vi "Init Screen.vi"(8 "error in":errorcluster) -> (0 "error out":errorcluster)   [LabVIEW 2020, in "Panther Dashboard.lvlib"]
uses:
  Panther Dashboard.lvlib
  Controls/Search.ctl
  Controls/Listbox.ctl
  Controls/Open Project.ctl
  Class/Project/Project.lvclass
panel:
  in  "Projects Opened":T1
  in  "Targets":T1
  out "Current Selection":string
  in  "Scan All":bool caption="Checkbox"
  in  "Include Dependencies":bool caption="Checkbox"
  in  "Scan Project":T2
  in  "Project history":T1
  in  "Open DQMH Project":T3
  # "Scanning a Project\n1. Select the Project and Target  where you want to work with Panther Dashboard\n2. Choose whether to scan the entire project or select specific modules to scan.\n3. Decide whether to include dependency modules in the scan.\n4. Click the Scan Project button."
  # "Working with previously Scanned Projects (Listed in Project History List):\n1. Double Click one of the Projects listed in the Project History\n\nWorking with previously Scanned Projects (not listed in the Project History)\n2. Click the Open DQMH Project and browse for your previously Scanned Project"
  # "1"
  # "1"
  # "1"
  # "2"
  # "4"
  # "2"
  # "3"
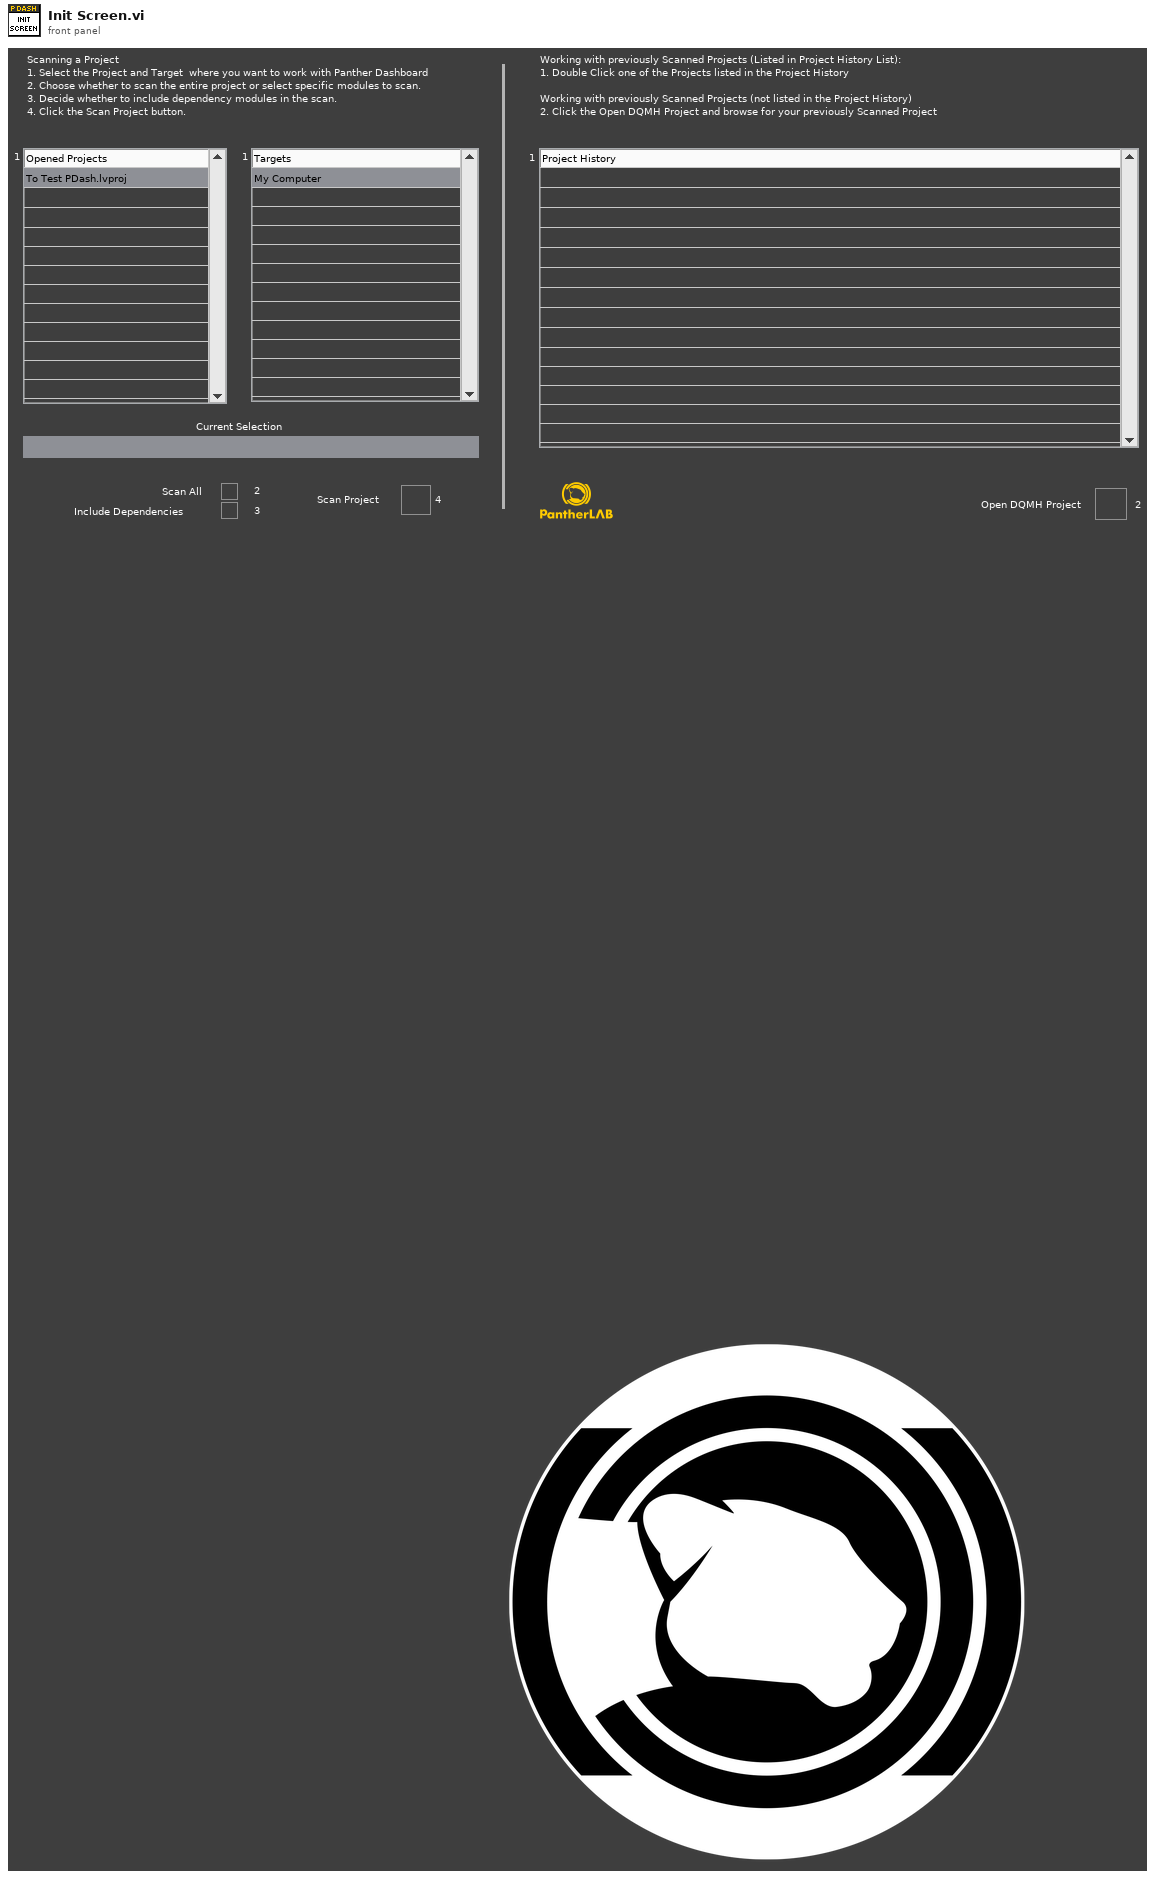
[diagram p1: front panel]
types:
  T1 = typedef "Listbox.ctl" = i32
  T2 = typedef "Search.ctl" = bool
  T3 = typedef "Open Project.ctl" = bool
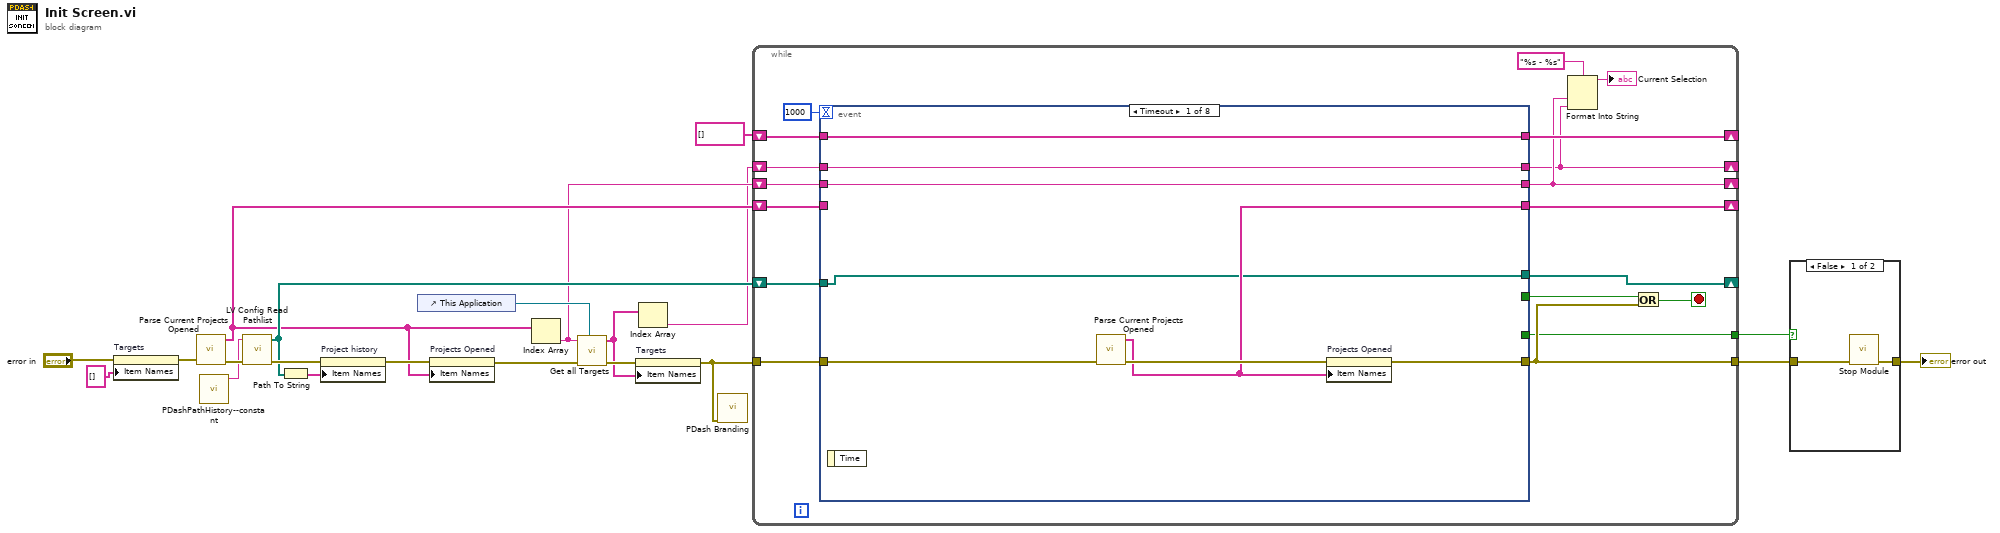
[diagram p0: block diagram]
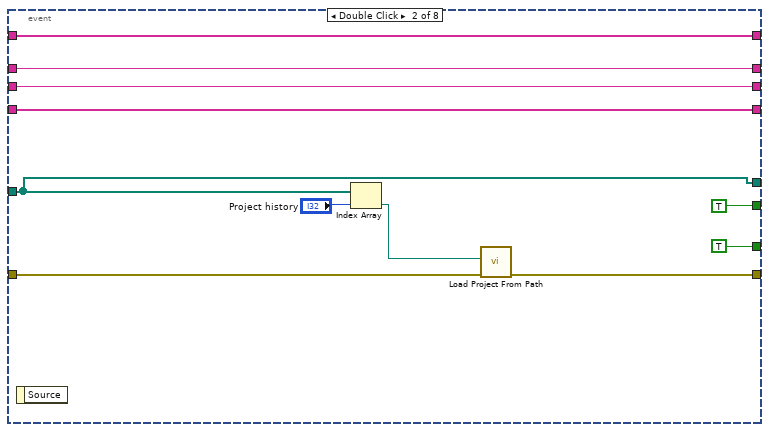
[diagram p2: hidden frame]
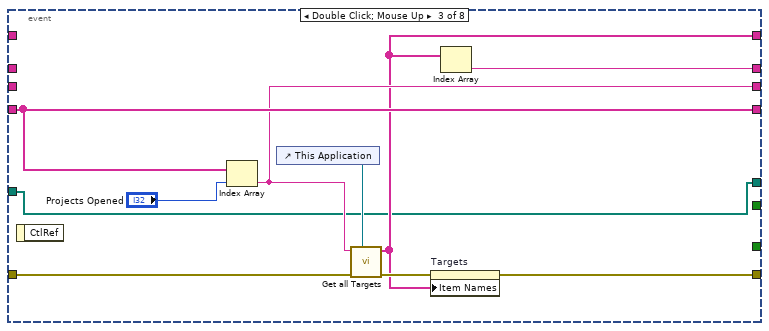
[diagram p3: hidden frame]
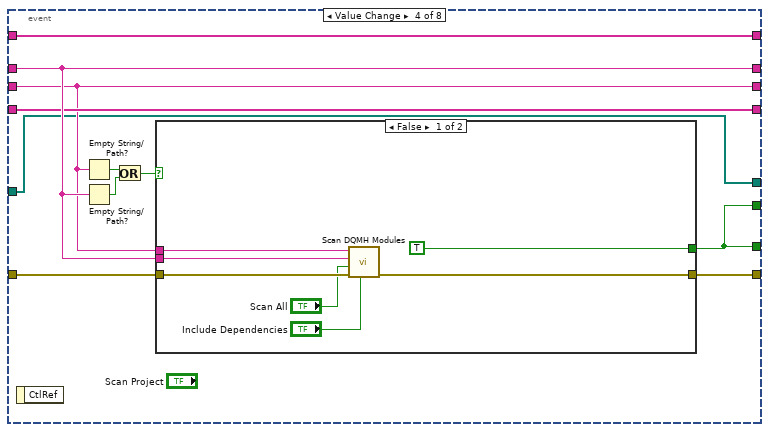
[diagram p4: hidden frame]
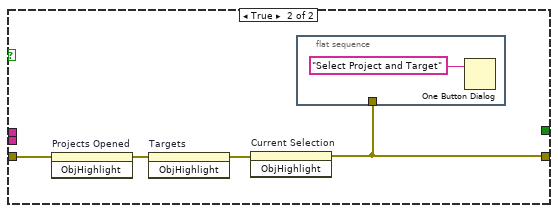
[diagram p5: hidden frame]
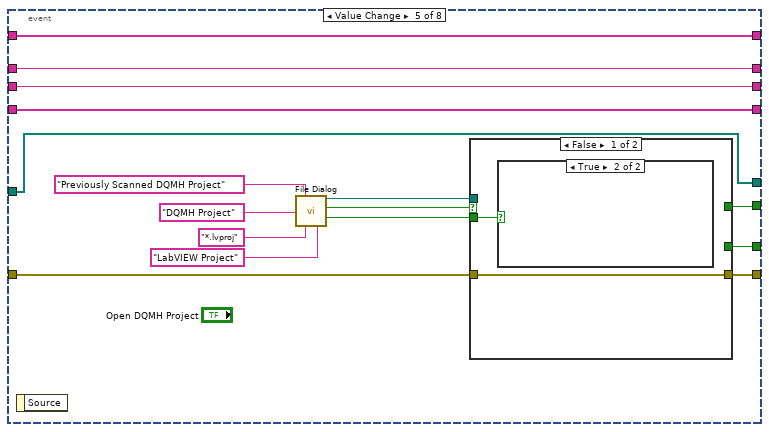
[diagram p6: hidden frame]
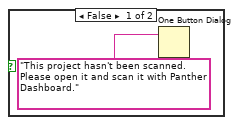
[diagram p7: hidden frame]
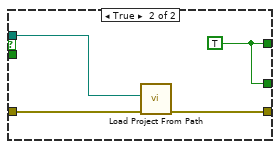
[diagram p8: hidden frame]
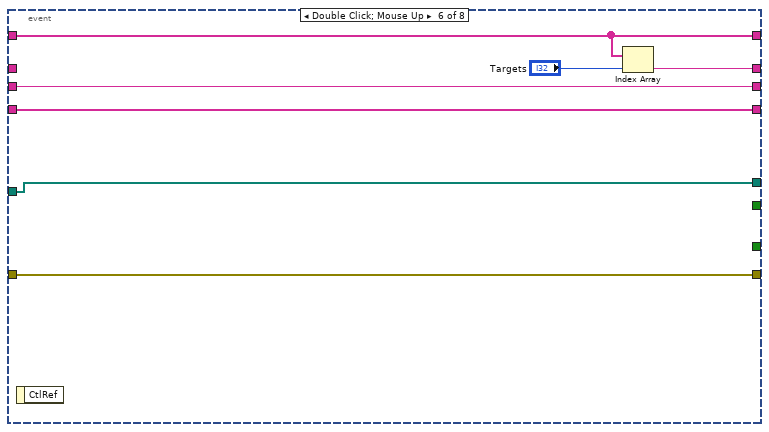
[diagram p9: hidden frame]
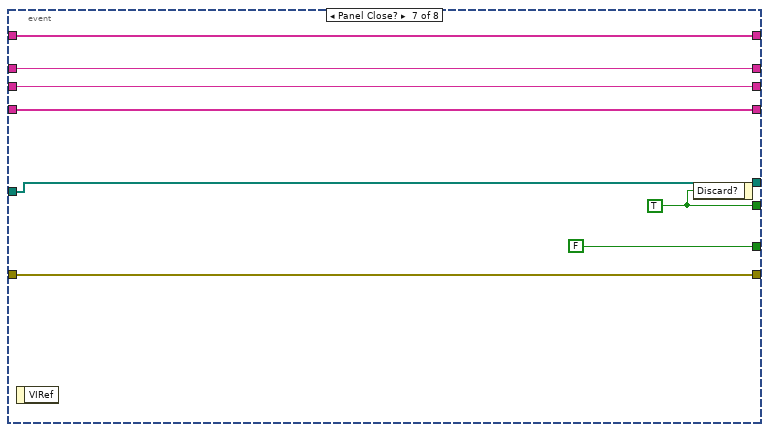
[diagram p10: hidden frame]
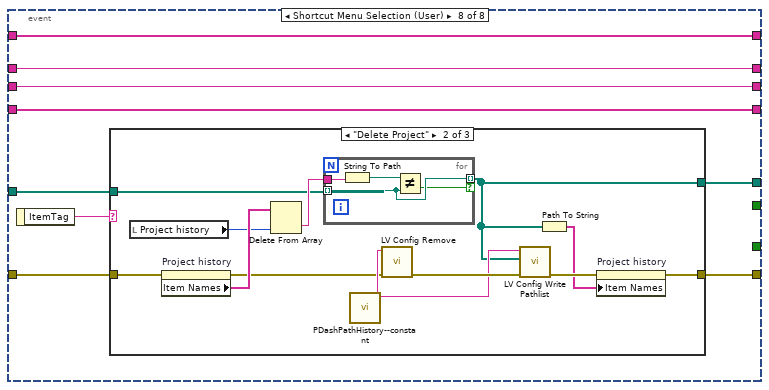
[diagram p11: hidden frame]
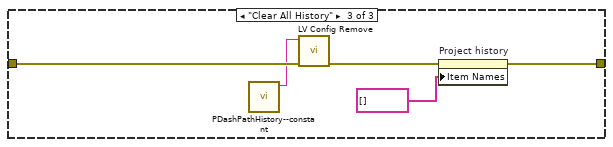
[diagram p13: hidden frame]
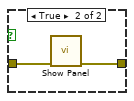
[diagram p14: hidden frame]
diagram:
  n1 = property on="Targets" class="LstBox (strict)"(error in="error in", "Item Names"=string[] []) -> (error out=w17:errorcluster)  [unwired: 1 in, 1 out]
  n2 = call "Parse Current Projects Opened.vi"("error in"=w17) -> ("error out"=w20:errorcluster, "Current Projects Opened"=w5:string[])  [unwired: 9 in]
  n3 = call "PDashPathHistory--constant.vi"() -> ("PDashPathHistory"=w12:string)  [unwired: 11 in]
  n4 = call <resource>:"LV Config Read Pathlist.vi"("error in"=w20, "key"=w12) -> ("error out"=w19:errorcluster, "value"=w11:path[])  [unwired: 3 in, 1 out]
  n5 = Path To String(path=w11) -> (string=w1:string[])
  n6 = property on="Project history" class="LstBox (strict)"(error in=w19, "Item Names"=w1) -> (error out=w18:errorcluster)  [unwired: 1 in, 1 out]
  n7 = control-ref of="This Application"() -> (w7:refnum<vi>)
  n8 = property on="Projects Opened" class="LstBox (strict)"(error in=w18, "Item Names"=w5) -> (error out=w14:errorcluster)  [unwired: 1 in, 1 out]
  n9 = Index Array(array=w5) -> (element=w4:string)  [unwired: 1 in]
  n10 = call "Get all Targets.vi"("App instance"=w7, "error in"=w14, "Project Selection"=w4) -> ("error out"=w15:errorcluster, "Targets"=w3:string[])  [unwired: 7 in]
  n11 = property on="Targets" class="LstBox (strict)"(error in=w15, "Item Names"=w3) -> (error out=w6:errorcluster)  [unwired: 1 in, 1 out]
  n12 = Index Array(array=w3) -> (element=w2:string)  [unwired: 1 in]
  n13 = call "PDash Branding.vi"("error in"=w6) -> ()  [unwired: 11 in]
  n14 = while {
    shift-right: [w34] -> _
    shift-left: string[] [] ("Targets") -> [w33]
    shift-right: [w25] -> _
    shift-left: w2 -> [w32]
    shift-right: [w26] -> _
    shift-left: w4 -> [w31]
    tunnel: [w28] -> w8
    shift-right: [w27] -> _
    shift-left: w5 -> [w35]
    tunnel: w6 -> [w39]
    tunnel: [w38] -> w21
    shift-right: [w23] -> _
    shift-left: w11 -> [w37]
    stop <- w29 stop-if-true
    n15 = event shown="[0] Timeout" {
      selector: _ -> [_ _ _ _ _ _ _ _]
      dyn-events: _ -> [_ _ _ _ _ _ _ _]
      timeout: 1000 -> [_ _ _ _ _ _ _ _]
      tunnel: w39 -> [w47 w58 w68 w79 w106 w121 w129 w138]
      tunnel: [w45 w57 w66 w78 w107 w121 w129 w137] -> w38
      tunnel: w37 -> [w40 w56 w59 w69 w92 w115 w122 w132]
      tunnel: [_ TRUE ("Discard?") _ w74 w101 _ w128 _] -> w36
      tunnel: w35 -> [_ w48 w65 w72 w102 w116 w123 w131]
      tunnel: [w44 w55 w61 w77 w105 w120 w127 w136] -> w34
      tunnel: w33 -> [w44 w55 _ w77 w105 w120 w127 w136]
      tunnel: [w43 w54 w60 w73 w104 w119 w126 w135] -> w25
      tunnel: w32 -> [w43 w54 _ w73 w104 _ w126 w135]
      tunnel: [w42 w53 w64 w71 w103 w118 w125 w134] -> w26
      tunnel: w31 -> [w42 w53 _ w71 w103 w118 w125 w134]
      tunnel: [_ TRUE ("Discard?") _ w74 w95 _ FALSE ("Discard?") _] -> w28
      tunnel: [w41 w48 w65 w72 w102 w116 w123 w131] -> w27
      tunnel: [w40 w56 w59 w69 w92 w115 w122 w130] -> w23
      event Timeout {
        n16 = event-data() -> ()  [unwired: 1 in, 1 out]
        n17 = call "Parse Current Projects Opened.vi"("error in"=w47) -> ("error out"=w46:errorcluster, "Current Projects Opened"=w41:string[])  [unwired: 9 in]
        n18 = property on="Projects Opened" class="LstBox (strict)"(error in=w46, "Item Names"=w41) -> (error out=w45:errorcluster)  [unwired: 1 in, 1 out]
      }
      event Double Click {
        n19 = event-data() -> ()  [unwired: 1 in, 1 out]
        n20 = Index Array(array=w56, index="Project history") -> (element=w51:path)
        n21 = call "Load Project From Path.vi"("error in"=w58, "Project Path"=w51) -> ("error out"=w57:errorcluster)  [unwired: 9 in]
      }
      event Double Click; Mouse Up {
        n22 = event-data() -> ()  [unwired: 1 in, 1 out]
        n23 = Index Array(array=w65, index="Projects Opened") -> (element=w64:string)
        n24 = control-ref of="This Application"() -> (w62:refnum<vi>)
        n25 = call "Get all Targets.vi"("App instance"=w62, "error in"=w68, "Project Selection"=w64) -> ("error out"=w67:errorcluster, "Targets"=w61:string[])  [unwired: 7 in]
        n26 = property on="Targets" class="LstBox (strict)"(error in=w67, "Item Names"=w61) -> (error out=w66:errorcluster)  [unwired: 1 in, 1 out]
        n27 = Index Array(array=w61) -> (element=w60:string)  [unwired: 1 in]
      }
      event Value Change {
        n28 = event-data() -> ()  [unwired: 1 in, 1 out]
        n29 = Empty String/Path?(string/path=w71) -> (empty?=w76:bool)
        n30 = Empty String/Path?(string/path=w73) -> (empty?=w70:bool)
        n31 = Or(x=w76, y=w70) -> (x .or. y?=w75:bool)
        n32 = case shown="False" w75 {
          tunnel: w79 -> [w86 w90]
          tunnel: [w85 w87] -> w78
          tunnel: w73 -> [w83 _]
          tunnel: w71 -> [w82 _]
          tunnel: [TRUE _] -> w74
          frame False {
            n33 = call "Scan DQMH Modules.vi"("Include Dependencies"="Include Dependencies", "error in"=w86, "Scan All"="Scan All", "Target"=w83, "Project"=w82) -> ("error out"=w85:errorcluster)  [unwired: 6 in]
          }
          frame True {
            n34 = invoke on="Projects Opened" class="LstBox (strict)" method="ObjHighlight"(error in=w90) -> (error out=w89:errorcluster)  [unwired: 2 in, 2 out]
            n35 = invoke on="Targets" class="LstBox (strict)" method="ObjHighlight"(error in=w89) -> (error out=w88:errorcluster)  [unwired: 2 in, 2 out]
            n36 = invoke on="Current Selection" class="Str" method="ObjHighlight"(error in=w88) -> (error out=w87:errorcluster)  [unwired: 2 in, 2 out]
            n37 = flat-sequence {
              tunnel: w87 -> [_]
              frame #0 {
                n38 = One Button Dialog(message="Select Project and Target") -> ()  [unwired: 1 in, 1 out]
              }
            }
          }
        }
      }
      event Value Change {
        n39 = event-data() -> ()  [unwired: 1 in, 1 out]
        n40 = call "File Dialog"("prompt"="Previously Scanned DQMH Project", "button label"="DQMH Project", "pattern (all files)"="*.lvproj", "pattern label"="LabVIEW Project") -> ("selected path"=w96:path, "exists"=w93:bool, "cancelled"=w94:bool)  [unwired: 8 in, 1 out]
        n41 = case shown="False" w93 {
          tunnel: w106 -> [w109 w114]
          tunnel: [w109 w113] -> w107
          tunnel: [_ w111] -> w101
          tunnel: w96 -> [_ w112]
          tunnel: [_ w111] -> w95
          tunnel: w94 -> [w108 _]
          frame False {
            n42 = case shown="True" w108 {
              frame False {
                n43 = One Button Dialog(message="This project hasn't been scanned. Please open it and scan it with Panther Dashboard.") -> ()  [unwired: 1 in, 1 out]
              }
              frame True {
              }
            }
          }
          frame True {
            w111 = TRUE
            n44 = call "Load Project From Path.vi"("error in"=w114, "Project Path"=w112) -> ("error out"=w113:errorcluster)  [unwired: 9 in]
          }
        }
      }
      event Double Click; Mouse Up {
        n45 = event-data() -> ()  [unwired: 1 in, 1 out]
        n46 = Index Array(array=w120, index="Targets") -> (element=w119:string)
      }
      event Panel Close? {
        w128 = TRUE ("Discard?")
        n47 = event-data() -> ()  [unwired: 1 in, 1 out]
        n48 = event-data("Discard?"=w128) -> ()  [unwired: 1 in, 1 out]
      }
      event Shortcut Menu Selection (User) {
        n49 = event-data() -> ("ItemTag"=w133:string)  [unwired: 1 in]
        n50 = case shown="\"Delete Project\"" w133 {
          tunnel: w138 -> [w139 w141 w160]
          tunnel: w132 -> [_ w143 _]
          tunnel: [w139 w149 w158] -> w137
          tunnel: [_ w142 _] -> w130
          frame Default {
          }
          frame "Delete Project" {
            n51 = local read "Project history"() -> (w146:T1)
            n52 = property on="Project history" class="LstBox (strict)"(error in=w141) -> (error out=w140:errorcluster, "Item Names"=w147:string[])  [unwired: 1 in, 1 out]
            n53 = Delete From Array(array=w147, index=w146) -> (deleted portion=w145:string)  [unwired: 1 in, 1 out]
            n54 = for {
              tunnel: w143 -> [w153] mode=indexing
              tunnel: w145 -> [w155]
              tunnel: [w153] -> w142 mode=indexing if=w152
              n55 = String To Path(string=w155) -> (path=w154:path)
              n56 = Not Equal?(x=w154, y=w153) -> (x != y?=w152:bool)
            }
            n57 = call "PDashPathHistory--constant.vi"() -> ("PDashPathHistory"=w148:string)  [unwired: 11 in]
            n58 = call <resource>:"LV Config Remove.vi"("error in"=w140, "key"=w148) -> ("error out"=w151:errorcluster)  [unwired: 5 in]
            n59 = call <resource>:"LV Config Write Pathlist.vi"("error in (no error)"=w151, "value"=w142, "key"=w148) -> ("error out"=w150:errorcluster)  [unwired: 4 in]
            n60 = Path To String(path=w142) -> (string=w144:string[])
            n61 = property on="Project history" class="LstBox (strict)"(error in=w150, "Item Names"=w144) -> (error out=w149:errorcluster)  [unwired: 1 in, 1 out]
          }
          frame "Clear All History" {
            n62 = call "PDashPathHistory--constant.vi"() -> ("PDashPathHistory"=w157:string)  [unwired: 11 in]
            n63 = call <resource>:"LV Config Remove.vi"("error in"=w160, "key"=w157) -> ("error out"=w159:errorcluster)  [unwired: 5 in]
            n64 = property on="Project history" class="LstBox (strict)"(error in=w159, "Item Names"=string[] []) -> (error out=w158:errorcluster)  [unwired: 1 in, 1 out]
          }
        }
      }
    }
    n65 = Format Into String(format string="%s - %s", w26, w25) -> (resulting string=→"Current Selection":string)  [unwired: 2 in, 1 out]
    n66 = Or(x=w36, y=w38) -> (x .or. y?=w29:bool)
  }
  n67 = case shown="False" w8 {
    tunnel: w21 -> [w162 w164]
    tunnel: [w161 w163] -> w13
    frame False {
      n68 = call "Stop Module.vi"("error in"=w162) -> ("error out"=w161:errorcluster)  [unwired: 10 in]
    }
    frame True {
      n69 = call "Show Panel.vi"("error in (no error)"=w164) -> ("error out"=w163:errorcluster)  [unwired: 10 in]
    }
  }
  "error out" <- w13
